vi "Test Fuzzy Control.vi"() -> ()   [LabVIEW 2020, in "NI_fuzzy logic.lvlib"]
doc: "This VI is designed as an example for building and testing a fuzzy controller application. It can be used as a general purpose Fuzzy Controller VI with up to four inputs and one output that can be interconnected to the desired process directly. After startup, the VI requests the fuzzy controller data file containing the fuzzy project data to be loaded from disk. You can enter input values using the input controls of the front panel when used as test environment. The controller output is also displayed on the front panel."
uses:
  <vilib>/addons/control/fuzzy/NI_fuzzy logic.lvlib
panel:
  out "maximums":dbl[](array[numeric]) format="%.2f"
  out "minimums":dbl[](array[numeric]) format="%.2f"
  in  "input value 4":dbl step=0.1 format="%.2f"
  out "input name 4":string
  in  "input value 3":dbl step=0.1 format="%.2f"
  out "input name 3":string
  in  "error ring":u16(ring)
  in  "stop":bool
  in  "input value 2":dbl step=0.1 format="%.2f"
  out "controller out":dbl format="%.2f"
  out "input name 2":string
  in  "input value 1":dbl step=0.1 format="%.2f"
  out "Controller":string
  out "output assessment":string="controlled result"
  out "input name 1":string
  # "Test environment for a \nFUZZY-CONTROLLER with up to four inputs"
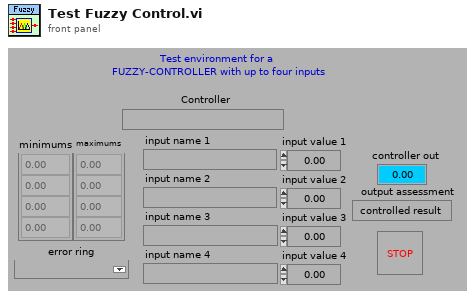
[diagram p1: front panel]
types:
  T1 = typedef "NI_fuzzy logic.lvlib/Fuzzy Datatype.ctl" = cluster{"Parameters":cluster{"antecedance":cluster{"ling.var.":string, "x-min":dbl, "x-max":dbl, "setarray":cluster{"linguistic term":string, "color":u32, "points":dbl[]}[]}[], "consequence":cluster{"ling.var.":string, "x-min":dbl, "x-max":dbl, "setarray":cluster{"linguistic term":string, "color":u32, "points":dbl[]}[]}[], "conclusions":u16[], "degree-of-support":dbl[], "defu":cluster{"inference":u16, "defumethod":u16, "modification":bool, "precision":u16, "no consequence":u16, "defaultvalue":dbl}[]}, "Description":cluster{"Info":cluster{"Path":path, "Controller Name":string, "Date":string, "Time":string}, "Author":string, "Description":string}}
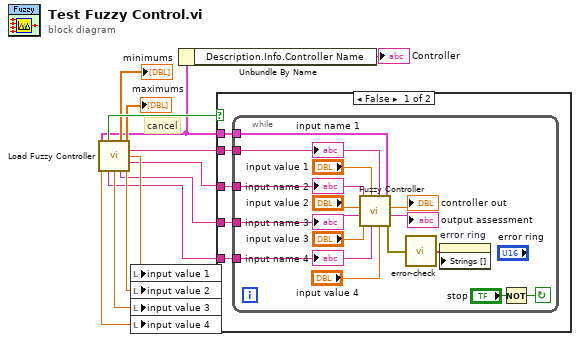
[diagram p0: block diagram]
diagram:
  # "cancel"
  n1 = call <vilib>:"Load Fuzzy Controller.vi"() -> ("Controller out"=w1:T1, "cancel"=w12:bool, "anteced. data range minimums"=→"minimums":dbl[], "anteced. data range maximums"=→"maximums":dbl[], "input name 1"=w7:string, "min 1"=w8:dbl, "input name 2"=w6:string, "min 4"=w11:dbl, "input name 4"=w4:string, "min 3"=w10:dbl, "input name 3"=w5:string, "min 2"=w9:dbl)  [unwired: 2 in, 2 out]
  n2 = local write "input value 1"(w8) -> ()
  n3 = local write "input value 2"(w9) -> ()
  n4 = local write "input value 3"(w10) -> ()
  n5 = local write "input value 4"(w11) -> ()
  n6 = Unbundle By Name(w1) -> ("Description.Info.Controller Name"=→"Controller":string)
  n7 = case shown="False" w12 {
    tunnel: w7 -> [w18 _]
    tunnel: w6 -> [w17 _]
    tunnel: w5 -> [w16 _]
    tunnel: w4 -> [w15 _]
    tunnel: w1 -> [w14 _]
    frame False {
      n8 = while {
        tunnel: w14 -> [w19]
        tunnel: w15 -> [w23]
        tunnel: w16 -> [w25]
        tunnel: w17 -> [w33]
        tunnel: w18 -> [w31]
        stop <- w21 continue-if-true
        n9 = call <vilib>:"Fuzzy Controller.vi"("Controller data"=w19, "in4"="input value 4", "name 1"=w31, "name 4"=w23, "in1"="input value 1", "in3"="input value 3", "name 3"=w25, "in2"="input value 2", "name 2"=w33) -> ("error-array"=w27:errorcluster[], "output assessment"=→"output assessment":string, "analog output"=→"controller out":dbl)
        n10 = call <vilib>:"error-check.vi"("error-array"=w27) -> ("error-strings"=w26:string[])
        n11 = property on="error ring" class="Ring (strict)"("Strings []"=w26) -> ()  [unwired: 2 in, 2 out]
        n12 = Not(x="stop") -> (.not. x?=w21:bool)
        "input name 2" <- w33
        "input name 1" <- w31
        "input name 3" <- w25
        "input name 4" <- w23
      }
    }
    frame True {
      # "The application quits\nsince the input file dialog\nrequesting for a Fuzzy Controller Data\nis cancelled.\nThis is just for security purposes\nbecause is makes no sense\nto run a Fuzzy Controller that is not parametrized."
    }
  }
